vi "initiate.vi"(0 "reference in":refnum<class "Test Controller.lvclass">, 5 "error in (no error)":errorcluster) -> (14 "reference out":refnum<class "Test Controller.lvclass">, 19 "error out":errorcluster)   [LabVIEW 2016, in "Test Controller.lvclass"]
uses:
  Test Controller.lvclass
  SYS/File Controller_llb/File Controller.lvclass
  SYS/Devices Controller_llb/Devices Controller.lvclass
  SYS/Items Controller_llb/Items Controller.lvclass
  GUI/GUI Controller_llb/GUI Controller.lvclass
  SYS/Notification Controller_class/Notification Controller.lvclass
  SYS/PartsTracking Controller_class/PartsTracking Controller.lvclass
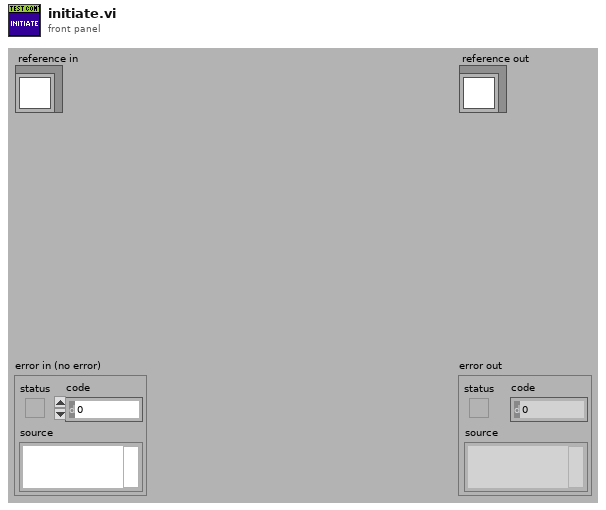
[diagram p1: front panel]
types:
  T1 = typedef "Test Controller.lvclass/ObjectAttributesRef.ctl" = refnum<data-value>
  T2 = typedef "Test Controller.lvclass/ObjectAttributes.ctl" = cluster{"MyAttribute":dbl, "Devices Controller_ref":refnum<class "Devices Controller.lvclass">, "File Controller_ref":refnum<class "File Controller.lvclass">, "Items Controller_ref":refnum<class "Items Controller.lvclass">, "GUI Controller_ref":refnum<class "GUI Controller.lvclass">, "NotificationController_ref":refnum<class "Notification Controller.lvclass">, "PartsTracking Controller_ref":refnum<class "PartsTracking Controller.lvclass">}
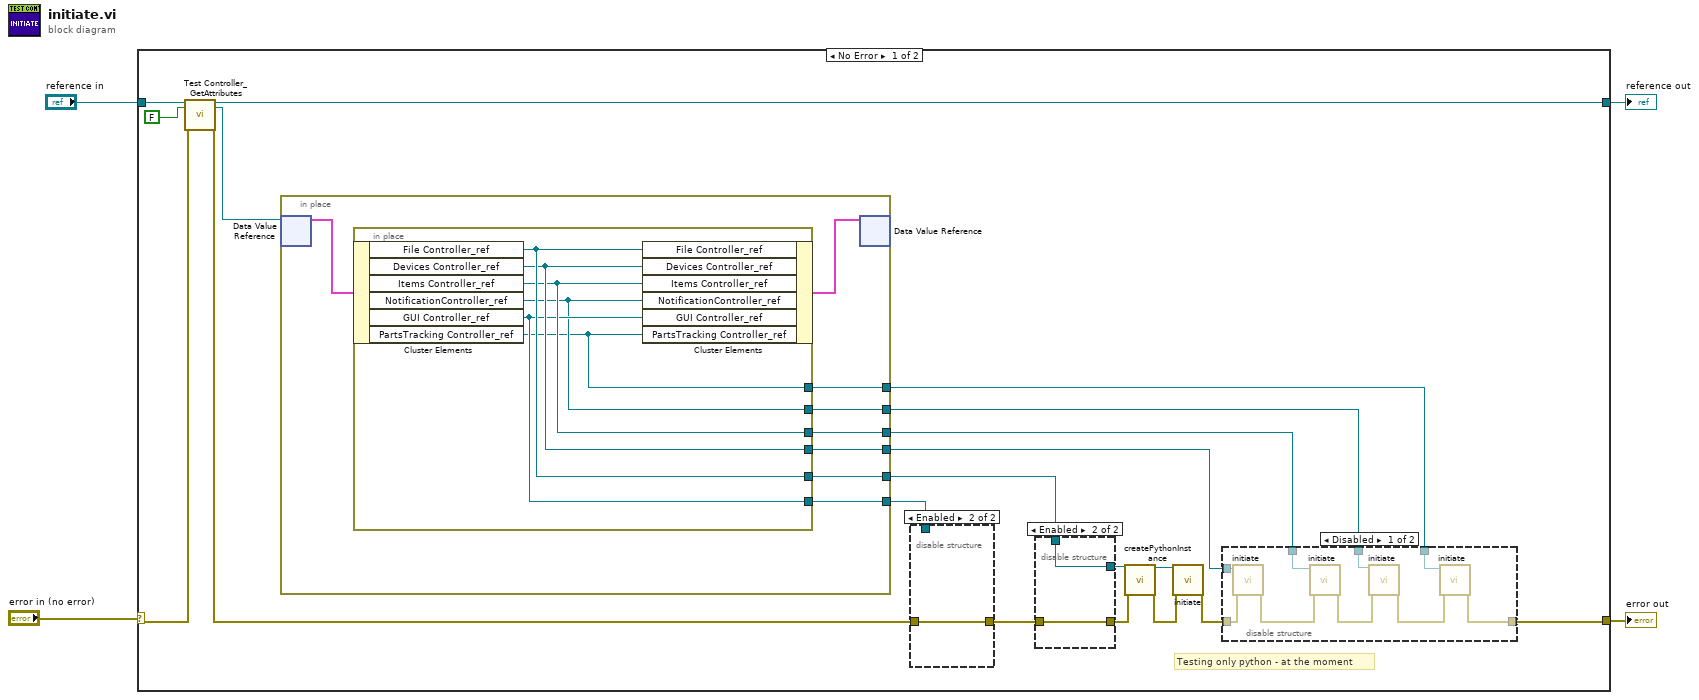
[diagram p0: block diagram]
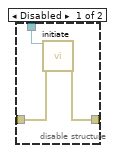
[diagram p2: hidden frame]
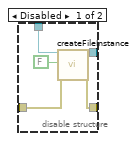
[diagram p4: hidden frame]
diagram:
  n1 = case shown="No Error" "error in (no error)" {
    selector: "error in (no error)" -> [w21 w60]
    tunnel: [w10 w60] -> w3
    tunnel: [w13 w59] -> w1
    tunnel: "reference in" -> [w23 w59]
    frame No Error {
      # "Testing only python - at the moment"
      n2 = call "Test Controller_GetAttributes.vi"("reference in"=w23, "return data? (T)"=FALSE, "error in (no error)"=w21) -> ("reference out"=w13:refnum<class "Test Controller.lvclass">, "attributes ref"=w20:T1, "error out"=w14:errorcluster)  [unwired: 13 in, 1 out]
      n3 = in-place {
        in-place-border: [w50] -> w12
        in-place-border: [w49] -> w19
        in-place-border: [w48] -> w17
        in-place-border: [w47] -> w16
        in-place-border: [w46] -> w15
        in-place-border: [w45] -> w11
        n4 = in-place-dvr #1(w20) -> (w51:T2)  [unwired: 1 out]
        n5 = in-place {
          in-place-border: [w58] -> w50
          in-place-border: [w57] -> w49
          in-place-border: [w56] -> w48
          in-place-border: [w55] -> w47
          in-place-border: [w54] -> w46
          in-place-border: [w53] -> w45
          n6 = in-place-cluster #2(w51) -> ("File Controller_ref"=w58:refnum<class "File Controller.lvclass">, "Devices Controller_ref"=w57:refnum<class "Devices Controller.lvclass">, "Items Controller_ref"=w56:refnum<class "Items Controller.lvclass">, "NotificationController_ref"=w54:refnum<class "Notification Controller.lvclass">, "GUI Controller_ref"=w55:refnum<class "GUI Controller.lvclass">, "PartsTracking Controller_ref"=w53:refnum<class "PartsTracking Controller.lvclass">)
          n7 = in-place-cluster #2("File Controller_ref"=w58, "Devices Controller_ref"=w57, "Items Controller_ref"=w56, "NotificationController_ref"=w54, "GUI Controller_ref"=w55, "PartsTracking Controller_ref"=w53) -> (w52:T2)
        }
        n8 = in-place-dvr #1(w52) -> ()  [unwired: 2 out]
      }
      n9 = disable-structure shown="Enabled" {
        disable-tunnel: w16 -> [w26 _]
        disable-tunnel: w14 -> [w25 w27]
        disable-tunnel: [w24 w27] -> w5
        frame Disabled {
          n10 = call "initiate.vi"("reference in"=w26, "error in (no error)"=w25) -> ("error out"=w24:errorcluster)  [unwired: 16 in, 1 out]
        }
        frame Enabled {
        }
      }
      n11 = disable-structure shown="Enabled" {
        disable-tunnel: w12 -> [w42 w43]
        disable-tunnel: [w41 w43] -> w9
        disable-tunnel: [w40 w44] -> w8
        disable-tunnel: w5 -> [w38 w44]
        frame Disabled {
          n12 = call "createFileInstance.vi"("reference in"=w42, "TSR?"=FALSE, "error in (no error)"=w38) -> ("reference out"=w41:refnum<class "File Controller.lvclass">, "error out"=w40:errorcluster)  [unwired: 15 in]
        }
        frame Enabled {
        }
      }
      n13 = call "createPythonInstance.vi"("reference in"=w9, "error in (no error)"=w8) -> ("reference out"=w6:refnum<class "File Controller.lvclass">, "error out"=w7:errorcluster)  [unwired: 16 in]
      n14 = call "initiate.vi"("reference in"=w6, "error in (no error)"=w7) -> ("error out"=w18:errorcluster)  [unwired: 16 in, 1 out]
      n15 = disable-structure shown="Disabled" {
        disable-tunnel: w19 -> [w36 _]
        disable-tunnel: w18 -> [w35 w37]
        disable-tunnel: w17 -> [w33 _]
        disable-tunnel: w15 -> [w32 _]
        disable-tunnel: w11 -> [w31 _]
        disable-tunnel: [w29 w37] -> w10
        frame Disabled {
          n16 = call "initiate.vi"("error in (no error)"=w35, "reference in"=w36) -> ("error out"=w34:errorcluster)  [unwired: 8 in, 1 out]
          n17 = call "initiate.vi"("error in (no error)"=w34, "reference in"=w33) -> ("error out"=w28:errorcluster)  [unwired: 8 in, 1 out]
          n18 = call "initiate.vi"("reference in"=w32, "error in (no error)"=w28) -> ("error out"=w30:errorcluster)  [unwired: 16 in, 1 out]
          n19 = call "initiate.vi"("error in (no error)"=w30, "reference in"=w31) -> ("error out"=w29:errorcluster)  [unwired: 8 in, 1 out]
        }
        frame Enabled {
        }
      }
    }
    frame Error {
    }
  }
  "error out" <- w3
  "reference out" <- w1
